vi "NumJacobian_X.vi"(4 "States":i32, 5 "F_FUNC":T1, 6 "Rows":i32, 7 "ExtraPassedData":variant, 10 "U":T2, 11 "X":T2) -> (0 "Error":bool, 3 "Result":T2)   [LabVIEW 2019, in "Trajectory_Library.lvlib"]
doc: "Creates a new LINEAR SYSTEM data cluster with the specified values. \n\n\nInputs: \n - XXX -- XXX.\n\nOutputs:\n - XXX -- XXX."
uses:
  Trajectory_Library.lvlib
  <vilib>/Analysis/Matrix/Datatypes/RealMatrix.ctl
  BiFunction_FUNC_TYPE.ctl
  <vilib>/Analysis/Matrix/Numeric/Subtract/Subtract - RM,RM.vi
  <vilib>/Analysis/Matrix/NI_Matrix.lvlib
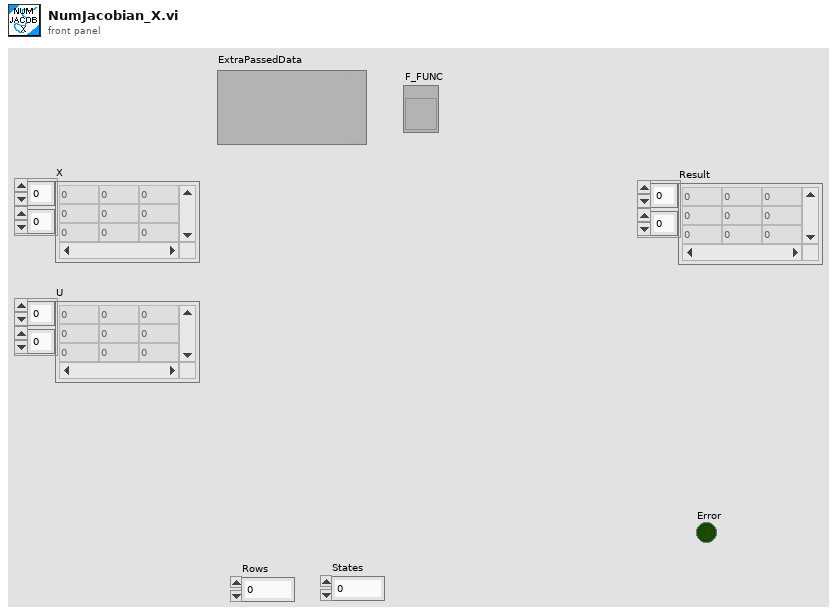
[diagram p1: front panel]
types:
  T1 = typedef "Trajectory_Library.lvlib/BiFunction_FUNC_TYPE.ctl" = refnum<vi>
  T2 = typedef "NI_Matrix.lvlib/RealMatrix.ctl" = dbl[][]
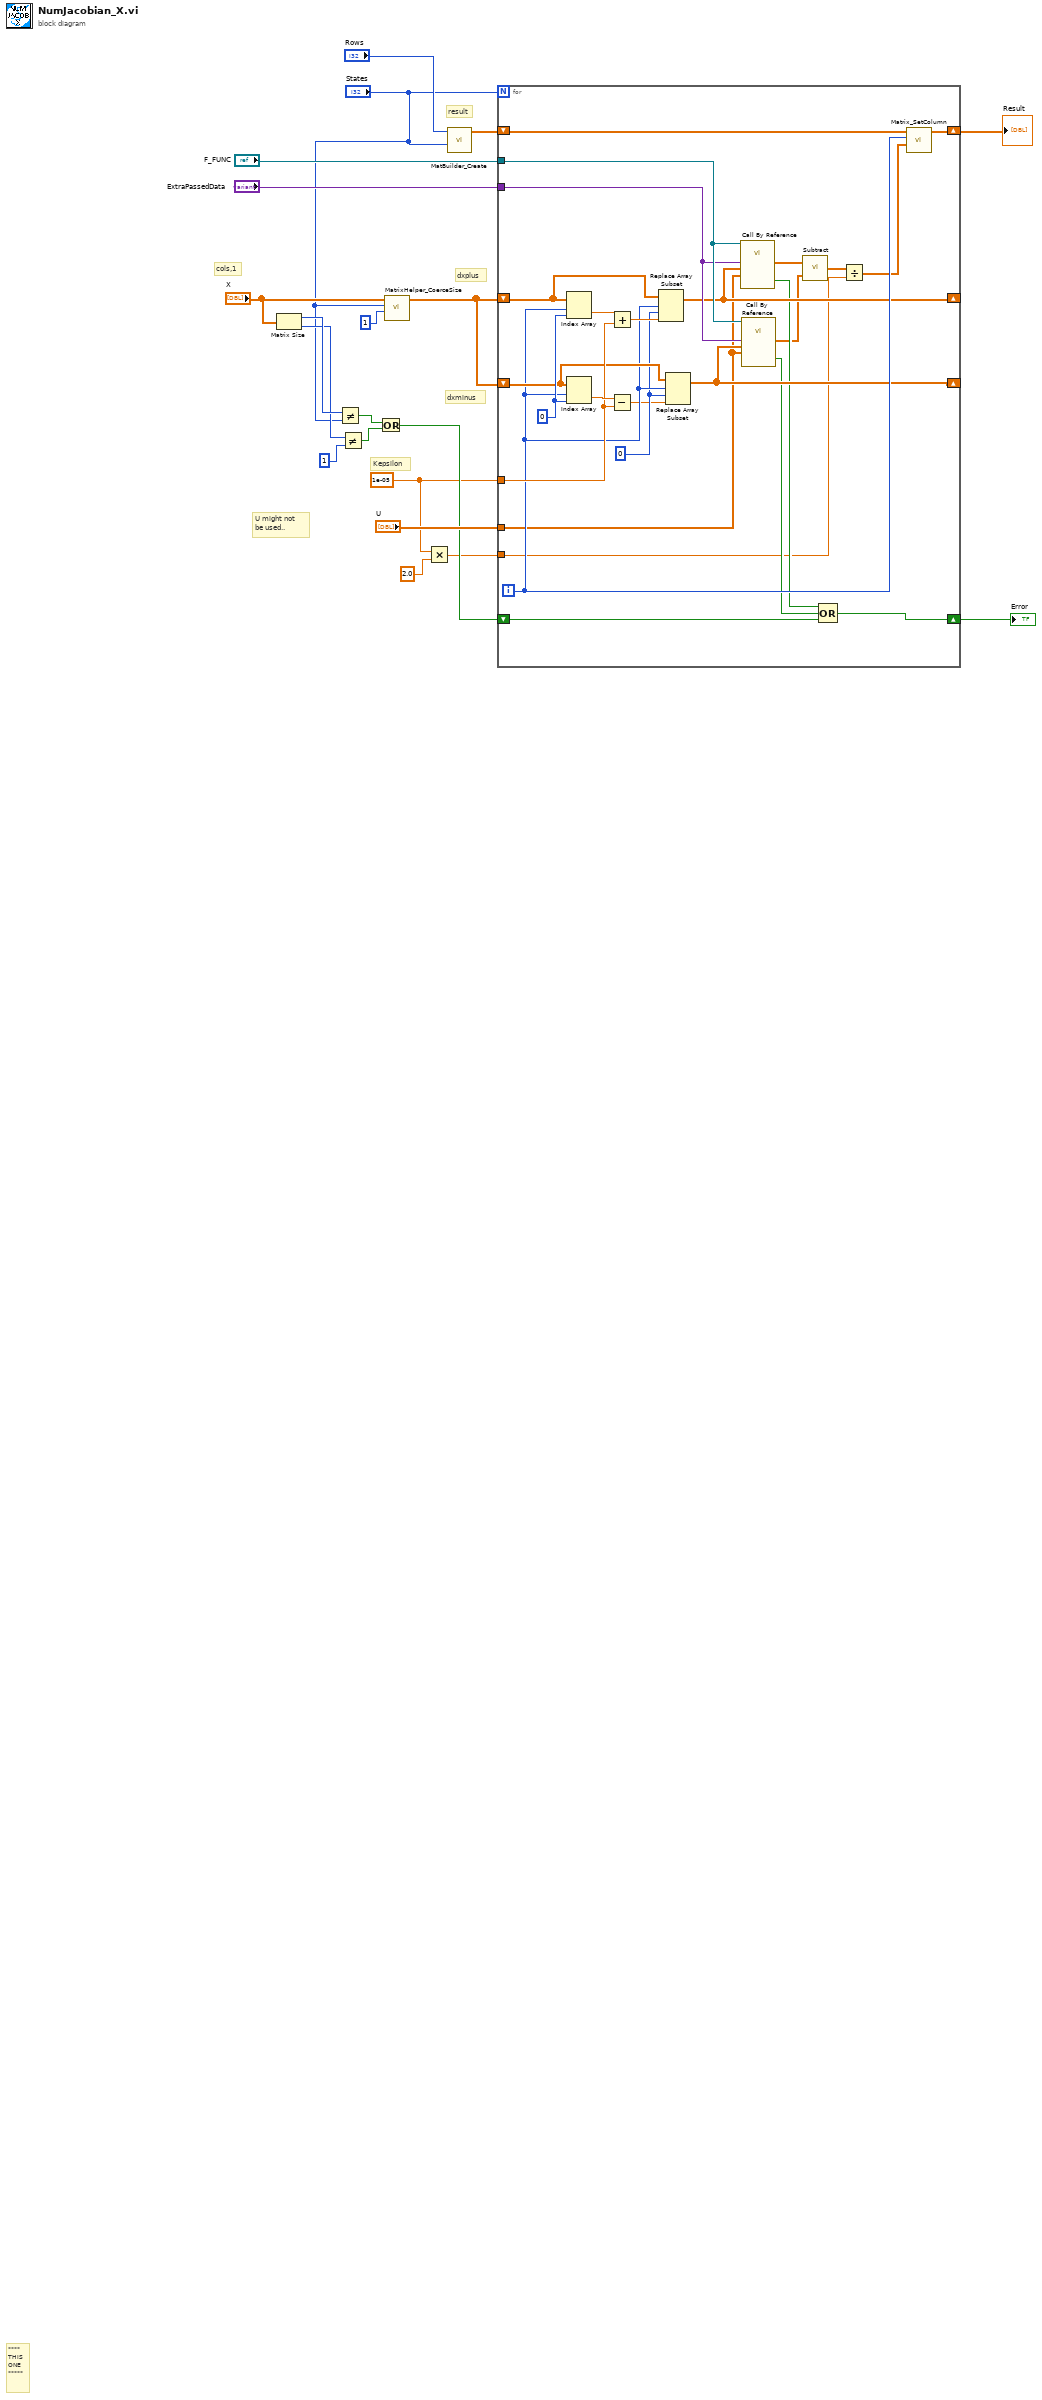
[diagram p0: block diagram]
diagram:
  w3 = 1e-05
  # "U might not \nbe used.."
  # "cols,1"
  # "dxminus"
  # "dxplus"
  # "Kepsilon"
  # "result"
  # "****\nTHIS\nONE\n*****"
  n1 = Matrix Size(0:"X") -> (1:w15:i32, 2:w14:i32)
  n2 = Not Equal?(x=w15, y="States") -> (x != y?=w8:bool)
  n3 = Not Equal?(x=w14, y=1) -> (x != y?=w7:bool)
  n4 = Or(x=w8, y=w7) -> (x .or. y?=w6:bool)
  n5 = call "MatrixHelper_CoerceSize.vi"("Columns"=1, "Rows"="States", "input matrix"="X") -> ("output matrix"=w11:T2)  [unwired: 8 in]
  n6 = Multiply(x=w3, y=2.0) -> (x*y=w4:dbl)
  n7 = call "MatBuilder_Create.vi"("Columns"="States", "Rows"="Rows") -> ("output matrix"=w19:T2)  [unwired: 9 in]
  n8 = for {
    N: "States" -> [_]
    tunnel: w3 -> [w39]
    shift-right: [w45] -> w1
    shift-left: w19 -> [w46]
    shift-right: [w32] -> _
    shift-left: w11 -> [w42]
    shift-right: [w31] -> _
    shift-left: w11 -> [w38]
    tunnel: "F_FUNC" -> [w34]
    tunnel: "ExtraPassedData" -> [w33]
    tunnel: "U" -> [w30]
    shift-right: [w28] -> w5
    shift-left: w6 -> [w29]
    tunnel: w4 -> [w22]
    i -> [w37]
    w36 = 0 ("disabled index (col)")
    w44 = 0 ("index (col)")
    n9 = Index Array(array=w42, index (row)=w37, index (col)=w44) -> (element=w43:dbl)
    n10 = Index Array(array=w38, index (row)=w37, index (col)=w44) -> (element=w40:dbl)
    n11 = Subtract(x=w40, y=w39) -> (x-y=w35:dbl)
    n12 = Add(x=w43, y=w39) -> (x+y=w41:dbl)
    n13 = Replace Array Subset(array=w42, new element=w41, index (row)=w37, index (col)=w36) -> (w32:T2)
    n14 = Replace Array Subset(array=w38, new element=w35, index (row)=w37, index (col)=w36) -> (w31:T2)
    n15 = call-by-ref "?"(reference=w34, "U"=w30, "X"=w32, "Variant"=w33) -> ("Error"=w26:bool, "NewX"=w25:T2)  [unwired: 8 in, 2 out]
    n16 = call-by-ref "?"(reference=w34, "U"=w30, "X"=w31, "Variant"=w33) -> ("Error"=w27:bool, "NewX"=w24:T2)  [unwired: 8 in, 2 out]
    n17 = call-poly <vilib>:"Subtract.vi"("Real Matrix B"=w24, "Real Matrix A"=w25) -> ("A - B"=w23:T2)
    n18 = Compound Arithmetic op=OR(w26, w27, w29) -> (w28:bool)
    n19 = Divide(x=w23, y=w22) -> (x/y=w21:T2)
    n20 = call "Matrix_SetColumn.vi"("Fill Vector"=w21, "Column"=w37, "input matrix"=w46) -> ("output matrix"=w45:T2)  [unwired: 8 in]
  }
  "Result" <- w1
  "Error" <- w5
